vi "Interface_Asset_Initalize Assets.vi"(8 "error in (no error)":errorcluster, 11 "Load in":refnum<class "Load.lvclass">) -> (0 "error out":errorcluster, 2 "TagDescriptions":refnum<class "tag descriptor.lvclass">[](array[class]), 3 "Load out":refnum<class "Load.lvclass">)   [LabVIEW 2015, in "Load.lvclass"]
uses:
  Load.lvclass
  <vilib>/NI/Tag Bus/tag/tag descriptor.lvclass
  TagBus/TagBus.lvclass
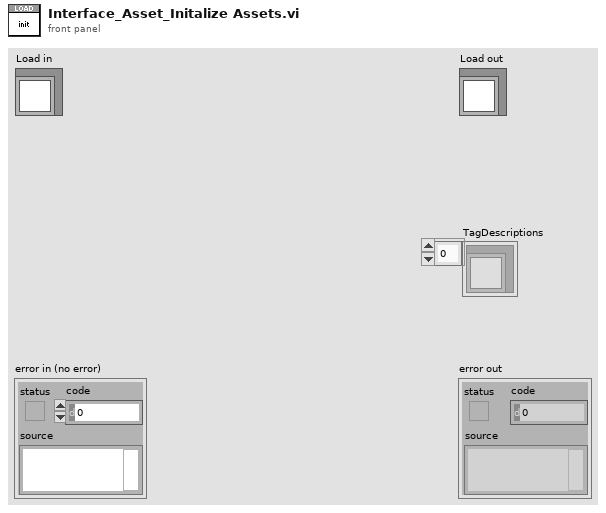
[diagram p1: front panel]
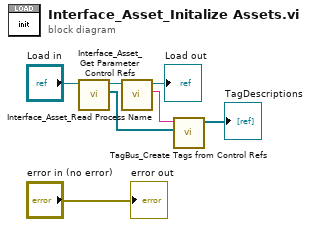
[diagram p0: block diagram]
diagram:
  n1 = call-dynamic "Interface_Asset_Get Parameter Control Refs.vi"("Load in"="Load in") -> ("Controls[]"=w1:refnum<vi>[], "Load out"=w2:refnum<class "Load.lvclass">)  [unwired: 8 in, 1 out]
  n2 = call-dynamic "Interface_Asset_Read Process Name.vi"("Load in"=w2) -> ("Process Name"=w6:string, "Load out"=→"Load out":refnum<class "Load.lvclass">)  [unwired: 9 in]
  n3 = call "TagBus_Create Tags from Control Refs.vi"("Array"=w1, "Prepend Tag Name"=w6) -> ("TagDescriptions"=→"TagDescriptions":refnum<class "tag descriptor.lvclass">[])  [unwired: 9 in]
  "error out" <- "error in (no error)"
